vi "UDP3LOOP.vi"(0 "Frequency, in Hz":dbl) -> ()   [LabVIEW 2009]
doc: "Pass information to global variables, and this vi will loop in the background (at a frequency which is set only once) and send the values over udp as a flattened strict time def.\nThis loop is stopped using the same global variable vi: UDP3GLOB has both the informational cluster, and the stop button.\nSister function is named UDP3read and it runs on the RT processor\nCheers!"
uses:
  UDP3GLOB.vi
panel:
  out "Heartbeat":bool
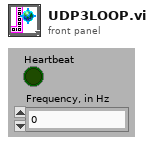
[diagram p1: front panel]
types:
  T1 = typedef "UDP 3.ctl" = cluster{"GPS":cluster{"Lat":dbl, "Longe":dbl}, "INS":cluster{"Compass":dbl, "Altitude":dbl, "Lat":dbl, "Longe":dbl}}
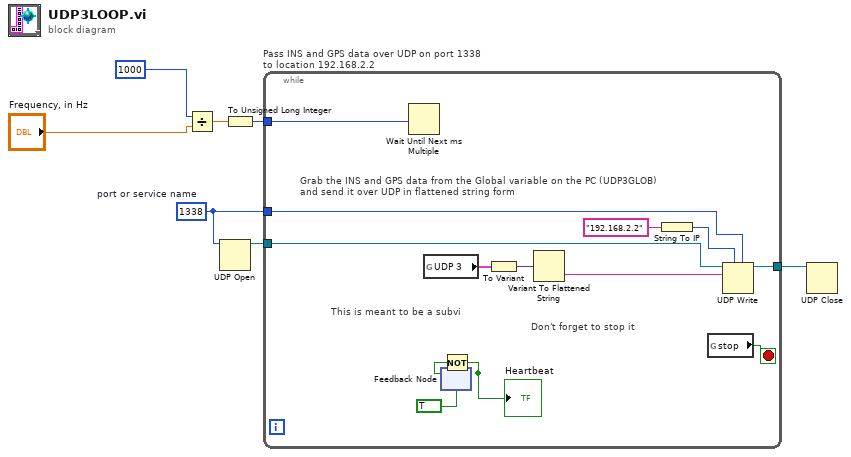
[diagram p0: block diagram]
diagram:
  w5 = u16 1338  # port or service name
  n1 = Divide(x=1000, y="Frequency, in Hz") -> (x/y=w2:dbl)
  n2 = UDP Open(11:w5) -> (port=w7:refnum<k16>)  [unwired: 4 in, 2 out]
  n3 = To Unsigned Long Integer(number=w2) -> (unsigned 32bit integer=w1:u32)
  n4 = while "Pass INS and GPS data over UDP on port 1338 to location 192.168.2.2" {
    tunnel: w7 -> [w20]
    tunnel: [w19] -> w6
    tunnel: w5 -> [w14]
    tunnel: w1 -> [w12]
    stop <- w13 stop-if-true
    # "Don't forget to stop it"
    # "This is meant to be a subvi"
    # "Grab the INS and GPS data from the Global variable on the PC (UDP3GLOB)\nand send it over UDP in flattened string form"
    n5 = Wait Until Next ms Multiple(millisecond multiple=w12) -> ()  [unwired: 1 out]
    n6 = global read "UDP3GLOB.vi" "UDP 3"() -> (w11:T1)
    n7 = feedback #1(TRUE) -> (w9:bool)
    n8 = Not(x=w9) -> (.not. x?=w8:bool)
    "Heartbeat" <- w8
    n9 = To Variant(anything=w11) -> (Variant=w16:variant)
    n10 = Variant To Flattened String(Variant=w16) -> (data string=w15:string)  [unwired: 1 out]
    n11 = String To IP(1:"192.168.2.2") -> (0:w17:u32)
    n12 = global read "UDP3GLOB.vi" "stop"() -> (w13:bool)
    n13 = UDP Write(address=w17, port or service name=w14, connection ID=w20, data in=w15) -> (3:w19:refnum<k16>)  [unwired: 2 in, 1 out]
  }
  n14 = UDP Close(connection ID=w6) -> ()  [unwired: 1 in, 2 out]
